vi "Yellow 1 to blue.vi"   [LabVIEW 2019]
uses:
  Global Var.vi
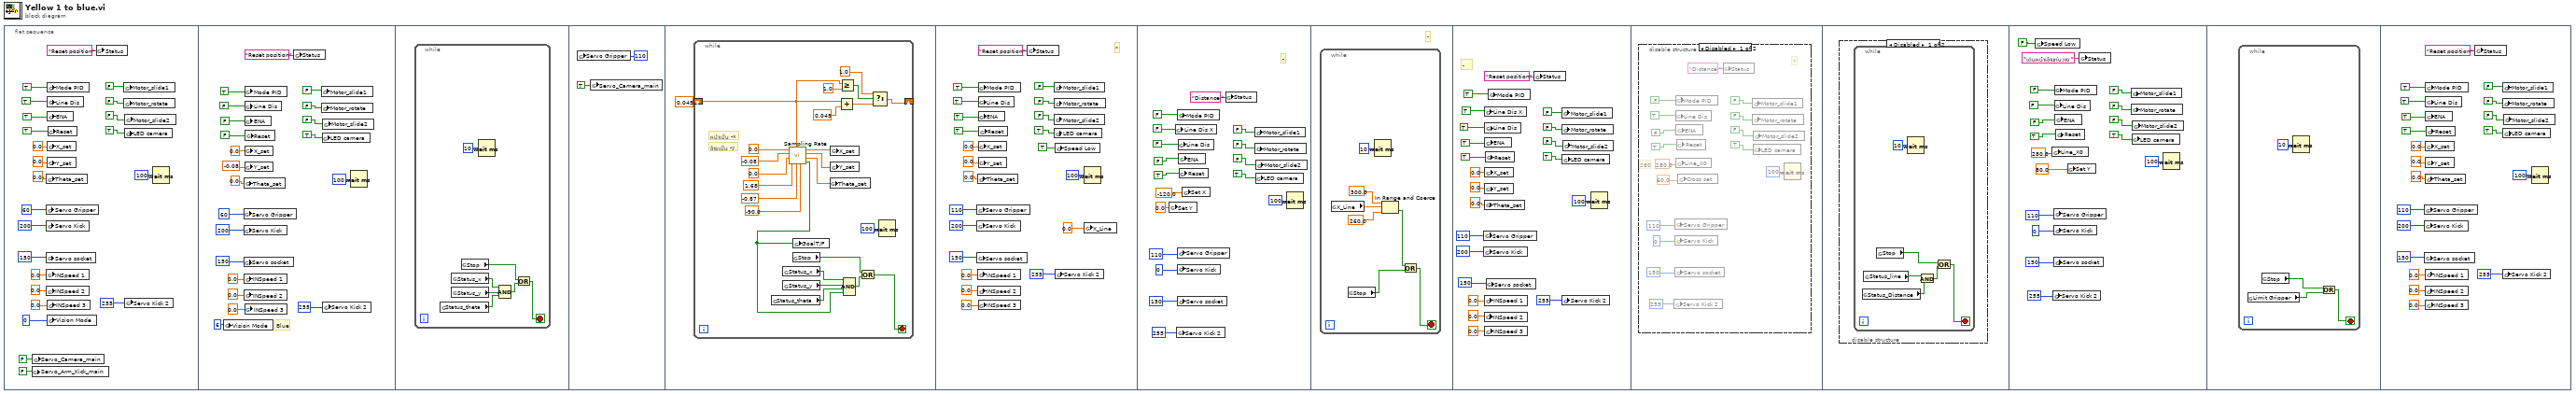
[diagram p0: block diagram]
diagram:
  n1 = flat-sequence {
    frame #0 {
      n2 = global write "Global Var.vi" "Servo_Arm_Kick_main"(FALSE ("Mode PID")) -> ()
      n3 = global write "Global Var.vi" "Servo_Camera_main"(FALSE ("Mode PID")) -> ()
      n4 = global write "Global Var.vi" "Servo Gripper"(u8 60 ("Servo Camera")) -> ()
      n5 = global write "Global Var.vi" "Servo Kick"(u8 200 ("Servo Camera")) -> ()
      n6 = global write "Global Var.vi" "Servo socket"(u8 150 ("Servo Camera")) -> ()
      n7 = global write "Global Var.vi" "Theta_set"(0.0 ("Theta_set")) -> ()
      n8 = global write "Global Var.vi" "INSpeed 1"(0.0 ("X_set")) -> ()
      n9 = global write "Global Var.vi" "INSpeed 2"(0.0 ("Y_set")) -> ()
      n10 = global write "Global Var.vi" "Mode PID"(TRUE ("Mode PID")) -> ()
      n11 = global write "Global Var.vi" "Line Dis"(TRUE ("Mode PID")) -> ()
      n12 = global write "Global Var.vi" "ENA"(TRUE ("ENA")) -> ()
      n13 = global write "Global Var.vi" "X_set"(0.0 ("X_set")) -> ()
      n14 = global write "Global Var.vi" "Y_set"(0.0 ("Y_set")) -> ()
      n15 = global write "Global Var.vi" "INSpeed 3"(0.0 ("Theta_set")) -> ()
      n16 = global write "Global Var.vi" "Vision Mode"(i16 0 ("Vision Mode")) -> ()
      n17 = global write "Global Var.vi" "Reset"(TRUE ("ENA")) -> ()
      n18 = global write "Global Var.vi" "Status"("Reset position" ("Status")) -> ()
      n19 = global write "Global Var.vi" "Motor_slide1"(FALSE ("Mode PID")) -> ()
      n20 = global write "Global Var.vi" "Motor_rotate"(FALSE ("ENA")) -> ()
      n21 = global write "Global Var.vi" "LED camera"(TRUE ("LED camera")) -> ()
      n22 = global write "Global Var.vi" "Motor_slide2"(FALSE ("ENA")) -> ()
      n23 = global write "Global Var.vi" "Servo Kick 2"(u8 255 ("Servo Camera")) -> ()
      n24 = Wait (ms)(milliseconds to wait=u32 100) -> ()  [unwired: 1 out]
    }
    frame #1 {
      # "Blue"
      n25 = global write "Global Var.vi" "Vision Mode"(i16 6 ("Vision Mode")) -> ()
      n26 = global write "Global Var.vi" "Servo Gripper"(u8 60 ("Servo Camera")) -> ()
      n27 = global write "Global Var.vi" "Servo Kick"(u8 200 ("Servo Camera")) -> ()
      n28 = global write "Global Var.vi" "Servo socket"(u8 150 ("Servo Camera")) -> ()
      n29 = global write "Global Var.vi" "Theta_set"(0.0 ("Theta_set")) -> ()
      n30 = global write "Global Var.vi" "INSpeed 1"(0.0 ("X_set")) -> ()
      n31 = global write "Global Var.vi" "INSpeed 2"(0.0 ("Y_set")) -> ()
      n32 = global write "Global Var.vi" "Mode PID"(TRUE ("Mode PID")) -> ()
      n33 = global write "Global Var.vi" "Line Dis"(FALSE ("Mode PID")) -> ()
      n34 = global write "Global Var.vi" "ENA"(FALSE ("ENA")) -> ()
      n35 = global write "Global Var.vi" "X_set"(0.0 ("X_set")) -> ()
      n36 = global write "Global Var.vi" "Y_set"(-0.08 ("Y_set")) -> ()
      n37 = global write "Global Var.vi" "INSpeed 3"(0.0 ("Theta_set")) -> ()
      n38 = global write "Global Var.vi" "Reset"(FALSE ("ENA")) -> ()
      n39 = global write "Global Var.vi" "Status"("Reset position" ("Status")) -> ()
      n40 = global write "Global Var.vi" "Motor_slide1"(FALSE ("Mode PID")) -> ()
      n41 = global write "Global Var.vi" "Motor_rotate"(FALSE ("ENA")) -> ()
      n42 = global write "Global Var.vi" "LED camera"(TRUE ("LED camera")) -> ()
      n43 = global write "Global Var.vi" "Motor_slide2"(FALSE ("ENA")) -> ()
      n44 = global write "Global Var.vi" "Servo Kick 2"(u8 255 ("Servo Camera")) -> ()
      n45 = Wait (ms)(milliseconds to wait=u32 100) -> ()  [unwired: 1 out]
    }
    frame #2 {
      n46 = while {
        stop <- w47 stop-if-true
        n47 = global read "Global Var.vi" "Status_theta"() -> (w49:bool)
        n48 = global read "Global Var.vi" "Status_x"() -> (w50:bool)
        n49 = global read "Global Var.vi" "Status_y"() -> (w51:bool)
        n50 = global read "Global Var.vi" "Stop"() -> (w45:bool)
        n51 = Wait (ms)(milliseconds to wait=u32 10) -> ()  [unwired: 1 out]
        n52 = Compound Arithmetic op=AND(w50, w51, w49) -> (w46:bool)
        n53 = Or(x=w45, y=w46) -> (x .or. y?=w47:bool)
      }
    }
    frame #3 {
      n54 = global write "Global Var.vi" "Servo Gripper"(u8 110 ("Servo Camera")) -> ()
      n55 = global write "Global Var.vi" "Servo_Camera_main"(TRUE ("Mode PID")) -> ()
    }
    frame #4 {
      n56 = while {
        shift-right: [w57] -> _
        shift-left: 0.045 -> [w55]
        stop <- w74 stop-if-true
        # "ซ้ายเป็น -y"
        # "หน้าเป็น -x"
        n57 = global read "Global Var.vi" "Status_theta"() -> (w76:bool)
        n58 = global read "Global Var.vi" "Status_x"() -> (w77:bool)
        n59 = global read "Global Var.vi" "Status_y"() -> (w78:bool)
        n60 = call "Sampling Rate.vi"("input a1"=-90.0, "input y1"=-0.87, "T(0-1)"=w55, "input x1"=1.68, "input a0"=0.0, "input y0"=-0.08, "input x0"=0.0) -> ("GoalT/F"=w62:bool, "a_output"=w69:dbl, "y_output"=w70:dbl, "x_output"=w71:dbl)  [unwired: 1 in]
        n61 = global read "Global Var.vi" "Stop"() -> (w72:bool)
        n62 = global write "Global Var.vi" "GoalT/F"(w62) -> ()
        n63 = global write "Global Var.vi" "Theta_set"(w69) -> ()
        n64 = global write "Global Var.vi" "X_set"(w71) -> ()
        n65 = global write "Global Var.vi" "Y_set"(w70) -> ()
        n66 = Add(x=w55, y=0.045) -> (x+y=w60:dbl)
        n67 = Greater Or Equal?(x=w55, y=1.0) -> (x >= y?=w59:bool)
        n68 = Compound Arithmetic op=AND(w77, w78, w76, w62) -> (w73:bool)
        n69 = Or(x=w72, y=w73) -> (x .or. y?=w74:bool)
        n70 = Select(t=1.0, s=w59, f=w60) -> (s? t:f=w57:dbl)
        n71 = Wait (ms)(milliseconds to wait=u32 100) -> ()  [unwired: 1 out]
      }
    }
    frame #5 {
      # "*"
      n72 = global write "Global Var.vi" "Servo Gripper"(u8 110 ("Servo Camera")) -> ()
      n73 = global write "Global Var.vi" "Servo Kick"(u8 200 ("Servo Camera")) -> ()
      n74 = global write "Global Var.vi" "Servo socket"(u8 150 ("Servo Camera")) -> ()
      n75 = global write "Global Var.vi" "Theta_set"(0.0 ("Theta_set")) -> ()
      n76 = global write "Global Var.vi" "INSpeed 1"(0.0 ("X_set")) -> ()
      n77 = global write "Global Var.vi" "INSpeed 2"(0.0 ("Y_set")) -> ()
      n78 = global write "Global Var.vi" "Mode PID"(TRUE ("Mode PID")) -> ()
      n79 = global write "Global Var.vi" "Line Dis"(TRUE ("Mode PID")) -> ()
      n80 = global write "Global Var.vi" "ENA"(TRUE ("ENA")) -> ()
      n81 = global write "Global Var.vi" "X_set"(0.0 ("X_set")) -> ()
      n82 = global write "Global Var.vi" "Y_set"(0.0 ("Y_set")) -> ()
      n83 = global write "Global Var.vi" "INSpeed 3"(0.0 ("Theta_set")) -> ()
      n84 = global write "Global Var.vi" "Reset"(TRUE ("ENA")) -> ()
      n85 = global write "Global Var.vi" "Status"("Reset position" ("Status")) -> ()
      n86 = global write "Global Var.vi" "Motor_slide1"(FALSE ("Mode PID")) -> ()
      n87 = global write "Global Var.vi" "Motor_rotate"(FALSE ("ENA")) -> ()
      n88 = global write "Global Var.vi" "Motor_slide2"(FALSE ("ENA")) -> ()
      n89 = global write "Global Var.vi" "LED camera"(TRUE ("LED camera")) -> ()
      n90 = global write "Global Var.vi" "Speed Low"(TRUE ("LED camera")) -> ()
      n91 = global write "Global Var.vi" "Servo Kick 2"(u8 255 ("Servo Camera")) -> ()
      n92 = Wait (ms)(milliseconds to wait=u32 100) -> ()  [unwired: 1 out]
      n93 = global write "Global Var.vi" "X_Line"(0.0 ("X_set")) -> ()
    }
    frame #6 {
      # "-"
      n94 = global write "Global Var.vi" "Set Y"(0.0 ("Y_set")) -> ()
      n95 = global write "Global Var.vi" "Line Dis X"(FALSE ("Mode PID")) -> ()
      n96 = global write "Global Var.vi" "Servo Kick 2"(u8 255 ("Servo Camera")) -> ()
      n97 = global write "Global Var.vi" "Mode PID"(FALSE ("Mode PID")) -> ()
      n98 = global write "Global Var.vi" "Servo Gripper"(u8 110 ("Servo Camera")) -> ()
      n99 = global write "Global Var.vi" "Servo Kick"(u8 0 ("Servo Camera")) -> ()
      n100 = global write "Global Var.vi" "Servo socket"(u8 150 ("Servo Camera")) -> ()
      n101 = global write "Global Var.vi" "Line Dis"(FALSE ("Mode PID")) -> ()
      n102 = global write "Global Var.vi" "ENA"(FALSE ("ENA")) -> ()
      n103 = global write "Global Var.vi" "Reset"(TRUE ("ENA")) -> ()
      n104 = global write "Global Var.vi" "Set X"(-120.0 ("Y_set")) -> ()
      n105 = global write "Global Var.vi" "Status"("Distance " ("Status")) -> ()
      n106 = global write "Global Var.vi" "Motor_slide1"(FALSE ("Mode PID")) -> ()
      n107 = global write "Global Var.vi" "Motor_rotate"(FALSE ("ENA")) -> ()
      n108 = global write "Global Var.vi" "LED camera"(TRUE ("LED camera")) -> ()
      n109 = global write "Global Var.vi" "Motor_slide2"(FALSE ("ENA")) -> ()
      n110 = Wait (ms)(milliseconds to wait=u32 100) -> ()  [unwired: 1 out]
    }
    frame #7 {
      # "-"
      n111 = while {
        stop <- w123 stop-if-true
        n112 = global read "Global Var.vi" "X_Line"() -> (w121:dbl)
        n113 = global read "Global Var.vi" "Stop"() -> (w122:bool)
        n114 = Wait (ms)(milliseconds to wait=u32 10) -> ()  [unwired: 1 out]
        n115 = In Range and Coerce(upper limit=300.0, x=w121, lower limit=260.0) -> (In Range?=w118:bool)  [unwired: 1 out]
        n116 = Or(x=w118, y=w122) -> (x .or. y?=w123:bool)
      }
    }
    frame #8 {
      # "-"
      n117 = global write "Global Var.vi" "Servo Gripper"(u8 110 ("Servo Camera")) -> ()
      n118 = global write "Global Var.vi" "Servo Kick"(u8 200 ("Servo Camera")) -> ()
      n119 = global write "Global Var.vi" "Line Dis X"(TRUE ("Mode PID")) -> ()
      n120 = global write "Global Var.vi" "Theta_set"(0.0 ("Theta_set")) -> ()
      n121 = global write "Global Var.vi" "INSpeed 1"(0.0 ("X_set")) -> ()
      n122 = global write "Global Var.vi" "INSpeed 2"(0.0 ("Y_set")) -> ()
      n123 = global write "Global Var.vi" "Line Dis"(TRUE ("Mode PID")) -> ()
      n124 = global write "Global Var.vi" "ENA"(TRUE ("ENA")) -> ()
      n125 = global write "Global Var.vi" "X_set"(0.0 ("X_set")) -> ()
      n126 = global write "Global Var.vi" "Y_set"(0.0 ("Y_set")) -> ()
      n127 = global write "Global Var.vi" "INSpeed 3"(0.0 ("Theta_set")) -> ()
      n128 = global write "Global Var.vi" "Reset"(TRUE ("ENA")) -> ()
      n129 = global write "Global Var.vi" "Servo socket"(u8 150 ("Servo Camera")) -> ()
      n130 = global write "Global Var.vi" "Mode PID"(TRUE ("Mode PID")) -> ()
      n131 = global write "Global Var.vi" "Status"("Reset position" ("Status")) -> ()
      n132 = global write "Global Var.vi" "Motor_slide1"(FALSE ("Mode PID")) -> ()
      n133 = global write "Global Var.vi" "Motor_rotate"(FALSE ("ENA")) -> ()
      n134 = global write "Global Var.vi" "Servo Kick 2"(u8 255 ("Servo Camera")) -> ()
      n135 = global write "Global Var.vi" "LED camera"(TRUE ("LED camera")) -> ()
      n136 = global write "Global Var.vi" "Motor_slide2"(FALSE ("ENA")) -> ()
      n137 = Wait (ms)(milliseconds to wait=u32 100) -> ()  [unwired: 1 out]
    }
    frame #9 {
      n138 = disable-structure shown="Disabled" {
        frame Disabled {
          # "280"
          # "*"
          n139 = global write "Global Var.vi" "Servo Kick 2"(u8 255 ("Servo Camera")) -> ()
          n140 = global write "Global Var.vi" "Servo Gripper"(u8 110 ("Servo Camera")) -> ()
          n141 = global write "Global Var.vi" "Servo Kick"(u8 0 ("Servo Camera")) -> ()
          n142 = global write "Global Var.vi" "Servo socket"(u8 150 ("Servo Camera")) -> ()
          n143 = global write "Global Var.vi" "Mode PID"(FALSE ("Mode PID")) -> ()
          n144 = global write "Global Var.vi" "Line Dis"(TRUE ("Mode PID")) -> ()
          n145 = global write "Global Var.vi" "ENA"(FALSE ("ENA")) -> ()
          n146 = global write "Global Var.vi" "Line_X0"(280.0 ("Y_set")) -> ()
          n147 = global write "Global Var.vi" "Reset"(TRUE ("ENA")) -> ()
          n148 = global write "Global Var.vi" "Cross set"(60.0 ("Y_set")) -> ()
          n149 = global write "Global Var.vi" "Status"("Distance " ("Status")) -> ()
          n150 = global write "Global Var.vi" "Motor_slide1"(FALSE ("Mode PID")) -> ()
          n151 = global write "Global Var.vi" "Motor_rotate"(FALSE ("ENA")) -> ()
          n152 = global write "Global Var.vi" "LED camera"(TRUE ("LED camera")) -> ()
          n153 = global write "Global Var.vi" "Motor_slide2"(FALSE ("ENA")) -> ()
          n154 = Wait (ms)(milliseconds to wait=u32 100) -> ()  [unwired: 1 out]
        }
        frame Enabled {
        }
      }
    }
    frame #10 {
      n155 = disable-structure shown="Disabled" {
        frame Disabled {
          n156 = while {
            stop <- w166 stop-if-true
            n157 = global read "Global Var.vi" "Status_Distance"() -> (w162:bool)
            n158 = global read "Global Var.vi" "Status_line"() -> (w163:bool)
            n159 = global read "Global Var.vi" "Stop"() -> (w165:bool)
            n160 = Wait (ms)(milliseconds to wait=u32 10) -> ()  [unwired: 1 out]
            n161 = And(x=w163, y=w162) -> (x .and. y?=w164:bool)
            n162 = Or(x=w165, y=w164) -> (x .or. y?=w166:bool)
          }
        }
        frame Enabled {
        }
      }
    }
    frame #11 {
      n163 = global write "Global Var.vi" "Speed Low"(FALSE ("LED camera")) -> ()
      n164 = global write "Global Var.vi" "Line_X0"(280.0 ("Y_set")) -> ()
      n165 = global write "Global Var.vi" "Servo Kick 2"(u8 255 ("Servo Camera")) -> ()
      n166 = global write "Global Var.vi" "Servo Gripper"(u8 110 ("Servo Camera")) -> ()
      n167 = global write "Global Var.vi" "Servo Kick"(u8 0 ("Servo Camera")) -> ()
      n168 = global write "Global Var.vi" "Servo socket"(u8 150 ("Servo Camera")) -> ()
      n169 = global write "Global Var.vi" "Mode PID"(FALSE ("Mode PID")) -> ()
      n170 = global write "Global Var.vi" "Line Dis"(FALSE ("Mode PID")) -> ()
      n171 = global write "Global Var.vi" "ENA"(FALSE ("ENA")) -> ()
      n172 = global write "Global Var.vi" "Reset"(TRUE ("ENA")) -> ()
      n173 = global write "Global Var.vi" "Set Y"(80.0 ("Y_set")) -> ()
      n174 = global write "Global Var.vi" "Status"("เดินหน้าเข้าแท่นวาง " ("Status")) -> ()
      n175 = global write "Global Var.vi" "Motor_slide1"(FALSE ("Mode PID")) -> ()
      n176 = global write "Global Var.vi" "Motor_rotate"(FALSE ("ENA")) -> ()
      n177 = global write "Global Var.vi" "LED camera"(TRUE ("LED camera")) -> ()
      n178 = global write "Global Var.vi" "Motor_slide2"(FALSE ("ENA")) -> ()
      n179 = Wait (ms)(milliseconds to wait=u32 100) -> ()  [unwired: 1 out]
    }
    frame #12 {
      n180 = while {
        stop <- w187 stop-if-true
        n181 = global read "Global Var.vi" "Limit Gripper"() -> (w185:bool)
        n182 = global read "Global Var.vi" "Stop"() -> (w186:bool)
        n183 = Wait (ms)(milliseconds to wait=u32 10) -> ()  [unwired: 1 out]
        n184 = Or(x=w186, y=w185) -> (x .or. y?=w187:bool)
      }
    }
    frame #13 {
      n185 = global write "Global Var.vi" "Servo Gripper"(u8 110 ("Servo Camera")) -> ()
      n186 = global write "Global Var.vi" "Servo Kick"(u8 200 ("Servo Camera")) -> ()
      n187 = global write "Global Var.vi" "Servo socket"(u8 150 ("Servo Camera")) -> ()
      n188 = global write "Global Var.vi" "Theta_set"(0.0 ("Theta_set")) -> ()
      n189 = global write "Global Var.vi" "INSpeed 1"(0.0 ("X_set")) -> ()
      n190 = global write "Global Var.vi" "INSpeed 2"(0.0 ("Y_set")) -> ()
      n191 = global write "Global Var.vi" "Mode PID"(TRUE ("Mode PID")) -> ()
      n192 = global write "Global Var.vi" "Line Dis"(TRUE ("Mode PID")) -> ()
      n193 = global write "Global Var.vi" "ENA"(TRUE ("ENA")) -> ()
      n194 = global write "Global Var.vi" "X_set"(0.0 ("X_set")) -> ()
      n195 = global write "Global Var.vi" "Y_set"(0.0 ("Y_set")) -> ()
      n196 = global write "Global Var.vi" "INSpeed 3"(0.0 ("Theta_set")) -> ()
      n197 = global write "Global Var.vi" "Reset"(TRUE ("ENA")) -> ()
      n198 = global write "Global Var.vi" "Status"("Reset position" ("Status")) -> ()
      n199 = global write "Global Var.vi" "Motor_slide1"(FALSE ("Mode PID")) -> ()
      n200 = global write "Global Var.vi" "Motor_rotate"(FALSE ("ENA")) -> ()
      n201 = global write "Global Var.vi" "Servo Kick 2"(u8 255 ("Servo Camera")) -> ()
      n202 = global write "Global Var.vi" "LED camera"(TRUE ("LED camera")) -> ()
      n203 = global write "Global Var.vi" "Motor_slide2"(FALSE ("ENA")) -> ()
      n204 = Wait (ms)(milliseconds to wait=u32 100) -> ()  [unwired: 1 out]
    }
  }
